vi "Enum枚举列表鼠标滚动事件.vi"(8 "error in (no error)":errorcluster caption="错误输入（无错误）", 9 "方向":enum16{"Horizontal", "Vertical"}(ring), 10 "Delta":i32, 11 "CtlRef":refnum<vi>) -> (0 "error out":errorcluster caption="错误输出", 3 "CtlRef 2":refnum<vi>)   [LabVIEW 2018]
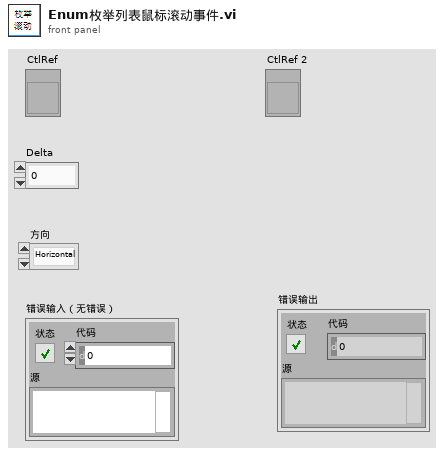
[diagram p1: front panel]
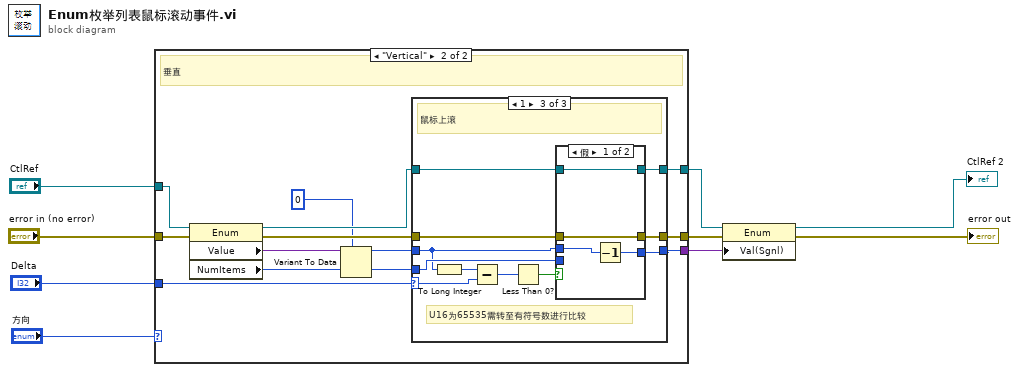
[diagram p0: block diagram]
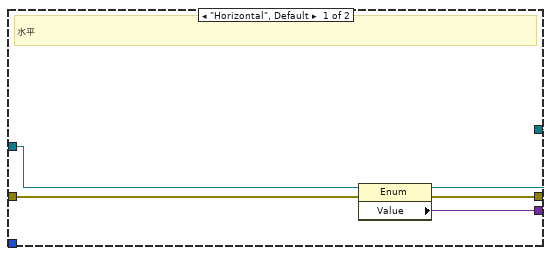
[diagram p2: hidden frame]
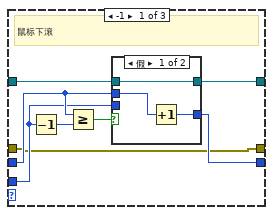
[diagram p3: hidden frame]
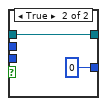
[diagram p4: hidden frame]
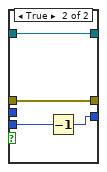
[diagram p6: hidden frame]
diagram:
  n1 = case shown="\"Vertical\"" "方向" {
    tunnel: "CtlRef" -> [w14 w26]
    tunnel: [w12 w24] -> w3
    tunnel: [w13 w23] -> w4
    tunnel: "Delta" -> [_ w21]
    tunnel: [w10 w20] -> w5
    tunnel: "error in (no error)" -> [w11 w18]
    frame "Horizontal", Default {
      # "水平"
      n2 = property class="Enum"(reference=w14, error in=w11) -> (reference out=w12:refnum<vi>, error out=w10:errorcluster, "Value"=w13:variant)
    }
    frame "Vertical" {
      # "垂直"
      n3 = property class="Enum"(reference=w26, error in=w18) -> (reference out=w25:refnum<vi>, error out=w19:errorcluster, "Value"=w17:variant, "NumItems"=w22:u32)
      n4 = Variant To Data(type=0, Variant=w17) -> (data=w15:i32)  [unwired: 1 in, 1 out]
      n5 = case shown="1" w21 {
        selector: w21 -> [_ _ w48]
        tunnel: w25 -> [w29 w42 w51]
        tunnel: w15 -> [w31 w41 w49]
        tunnel: [w33 w42 w52] -> w24
        tunnel: [w32 w41 w53] -> w23
        tunnel: w22 -> [w30 _ w50]
        tunnel: [w27 w40 w44] -> w20
        tunnel: w19 -> [w27 w40 w43]
        frame -1 {
          # "鼠标下滚"
          n6 = Decrement(x=w30) -> (x-1=w28:u32)
          n7 = Greater Or Equal?(x=w31, y=w28) -> (x >= y?=w34:bool)
          n8 = case shown="假" w34 {
            tunnel: w31 -> [w37 _]
            tunnel: [w36 u16 0] -> w32
            tunnel: [w35 w38] -> w33
            tunnel: w30 -> [_ _]
            tunnel: w29 -> [w35 w38]
            frame False {
              n9 = Increment(x=w37) -> (x+1=w36:i32)
            }
            frame True {
            }
          }
        }
        frame 0, Default {
        }
        frame 1 {
          # "U16为65535需转至有符号数进行比较"
          # "鼠标上滚"
          n10 = To Long Integer(number=w49) -> (32bit integer=w45:i32)
          n11 = Subtract(x=w45, y=w48) -> (x-y=w46:i32)
          n12 = Less Than 0?(x=w46) -> (x < 0?=w47:bool)
          n13 = case shown="假" w47 {
            tunnel: w51 -> [w57 w61]
            tunnel: w49 -> [w56 _]
            tunnel: [w55 w60] -> w53
            tunnel: [w57 w61] -> w52
            tunnel: w50 -> [_ w59]
            tunnel: [w54 w58] -> w44
            tunnel: w43 -> [w54 w58]
            frame False {
              n14 = Decrement(x=w56) -> (x-1=w55:i32)
            }
            frame True {
              n15 = Decrement(x=w59) -> (x-1=w60:u32)
            }
          }
        }
      }
    }
  }
  n16 = property class="Enum"(reference=w3, error in=w5, "Val(Sgnl)"=w4) -> (reference out=→"CtlRef 2":refnum<vi>, error out=→"error out":errorcluster)
